vi "Piston_Fire.vi"(10 "Fire?":bool) -> ()   [LabVIEW 2019]
uses:
  <vilib>/Rock Robotics/WPI/Solenoid/WPI_SolenoidValue.ctl
  <vilib>/Rock Robotics/WPI/Solenoid/WPI_SolenoidSetEnum.vi
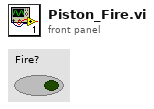
[diagram p1: front panel]
types:
  T1 = typedef "WPI_SolenoidDevRef.ctl" = cluster{"DevStatus":errorcluster, "Pneumatics Control Module":u8, "Forward Solenoid Channel":T2, "Reverse Solenoid Channel":T2}
  T2 = typedef "WPI_SolenoidChannel.ctl" = enum8{"Solenoid 0", "Solenoid 1", "Solenoid 2", "Solenoid 3", "Solenoid 4", "Solenoid 5", "Solenoid 6", "Solenoid 7", "Invalid"}
  T3 = typedef "WPI_SolenoidValue.ctl" = enum16{"Off", "On", "Forward", "Reverse"}
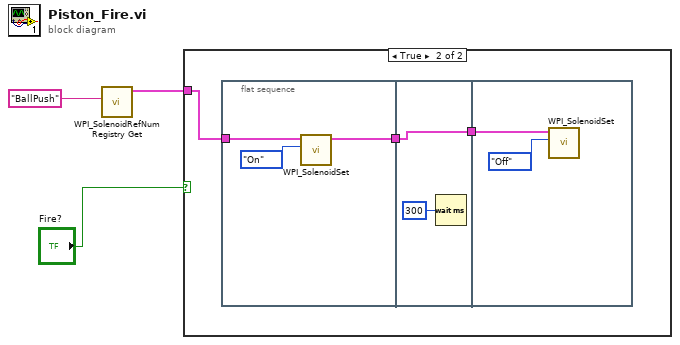
[diagram p0: block diagram]
diagram:
  n1 = call <vilib>:"WPI_SolenoidRefNum Registry Get.vi"("refnum name"="BallPush") -> ("SolenoidDevRef"=w1:T1)  [unwired: 9 in, 1 out]
  n2 = case shown="True" "Fire?" {
    tunnel: w1 -> [_ w6]
    frame False {
    }
    frame True {
      n3 = flat-sequence {
        tunnel: w6 -> [w9]
        tunnel: [w8] -> w5
        tunnel: w5 -> [w11]
        tunnel: [w11] -> w4
        tunnel: w4 -> [w13]
        frame #0 {
          n4 = call-poly <vilib>:"WPI_SolenoidSet.vi"("Value"=WPI_SolenoidValue."On", "SolenoidDevRef"=w9) -> ("SolenoidDevRef"=w8:T1)  [unwired: 8 in, 1 out]
        }
        frame #1 {
          n5 = Wait (ms)(milliseconds to wait=u32 300) -> ()  [unwired: 1 out]
        }
        frame #2 {
          n6 = call-poly <vilib>:"WPI_SolenoidSet.vi"("Value"=WPI_SolenoidValue."Off", "SolenoidDevRef"=w13) -> ()  [unwired: 8 in, 2 out]
        }
      }
    }
  }
